vi "AIT 664 - Add Data Channel.vi"(8 "error in (no error)":errorcluster, 11 "Node Ptr":u64 format="%.0x") -> (0 "error out":errorcluster)   [LabVIEW 2013, in "AIT 664 Custom Device.lvlib"]
doc: "Adds a single data channel to a 664 port"
uses:
  AIT 664 Custom Device.lvlib
  <vilib>/NI Veristand/Custom Device API/Custom Device Channel.ctl
  <vilib>/NI Veristand/Custom Device API/Custom Device Channel Type.ctl
  Controls/664 -Param.ctl
  Controls and Global/Global.vi
  <vilib>/NI Veristand/Custom Device API/Get Item Property (U32).vi
  <vilib>/NI Veristand/Custom Device API/Get Item Property (U32 Array).vi
  <vilib>/NI Veristand/Custom Device API/Get Item Property (Boolean).vi
  <vilib>/NI Veristand/Custom Device API/Custom Device API.lvlib
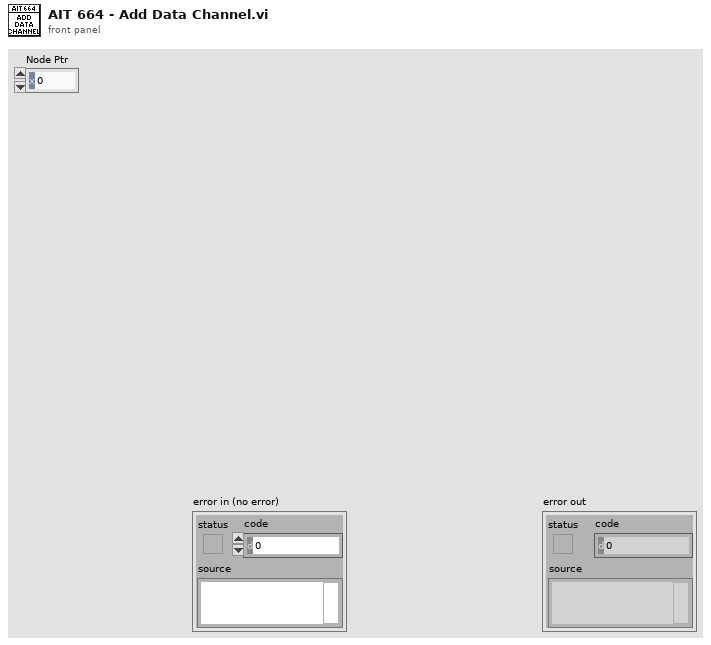
[diagram p1: front panel]
types:
  T1 = typedef "Custom Device API.lvlib/Custom Device Channel Type.ctl" = enum16{"Input", "Output"}
  T2 = typedef "AIT 664 Custom Device.lvlib/664 -Param.ctl" = cluster{"name":string, "firstByte":i32, "startBit":i32, "numberBits":i32, "scaleFactor":dbl, "scaleOffset":dbl, "signed":bool}
  T3 = typedef "Custom Device API.lvlib/Custom Device Channel.ctl" = cluster{"Type":T1, "Units":string, "Default Value":dbl, "Faultable":bool, "Scalable":bool}
  T4 = typedef "Custom Device API.lvlib/Custom Device Item Ref.ctl" = u64
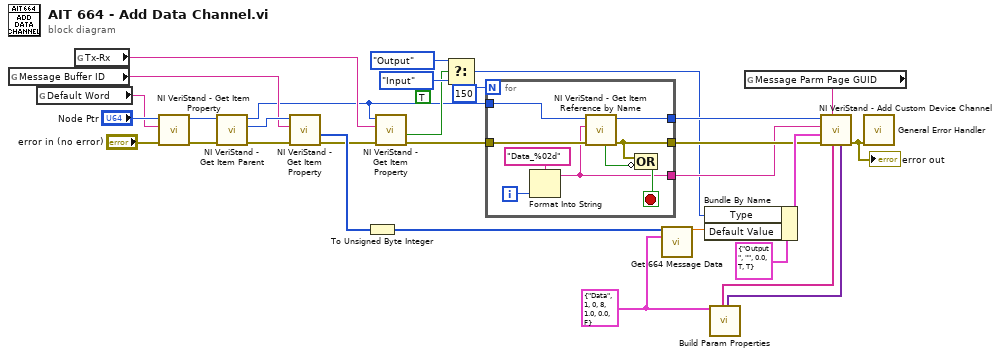
[diagram p0: block diagram]
diagram:
  (unwired) TRUE ("s")
  w9 = T2 {"name"="Data", "firstByte"=1, "startBit"=0, "numberBits"=8, "scaleFactor"=1.0, "scaleOffset"=0.0, "signed"=FALSE} ("1553 Parameter")
  n1 = global read "Global.vi" "Message Buffer ID"() -> (w19:string)
  n2 = global read "Global.vi" "Default Word"() -> (w24:string)
  n3 = global read "Global.vi" "Tx-Rx"() -> (w14:string)
  n4 = call-poly <vilib>:"NI VeriStand - Get Item Property.vi"("error in (no error)"="error in (no error)", "Property Name"=w24, "Item Ref in"="Node Ptr") -> ("error out"=w26:errorcluster, "Item Ref out"=w27:T4)  [unwired: 5 in, 2 out]
  n5 = call <vilib>:"NI VeriStand - Get Item Parent.vi"("error in (no error)"=w26, "Item Ref in"=w27) -> ("error out"=w20:errorcluster, "Parent Ref"=w21:T4, "Item Ref out"=w1:T4)  [unwired: 6 in, 1 out]
  n6 = call-poly <vilib>:"NI VeriStand - Get Item Property.vi"("error in (no error)"=w20, "Property Name"=w19, "Item Ref in"=w21) -> ("error out"=w15:errorcluster, "Value"=w18:u32[])  [unwired: 5 in, 2 out]
  n7 = To Unsigned Byte Integer(number=w18) -> (unsigned 8bit integer=w17:u8[])
  n8 = call-poly <vilib>:"NI VeriStand - Get Item Property.vi"("error in (no error)"=w15, "Property Name"=w14, "Item Ref in"=w1) -> ("error out"=w8:errorcluster, "Value"=w2:bool)  [unwired: 5 in, 2 out]
  n9 = Select(t=Custom_Device_Channel_Type."Output" ("Type"), s=w2, f=Custom_Device_Channel_Type."Input" ("Type")) -> (s? t:f=w3:T1)
  n10 = for {
    N: 150 -> [_]
    tunnel: w1 -> [w39]
    tunnel: w8 -> [w38]
    tunnel: [w36] -> w7
    tunnel: [w34] -> w6
    tunnel: [w31] -> w5
    i -> [w33]
    stop <- w37 stop-if-true
    n11 = Format Into String(format string="Data_%02d" ("name"), w33) -> (resulting string=w31:string)  [unwired: 2 in, 1 out]
    n12 = call <vilib>:"NI VeriStand - Get Item Reference by Name.vi"("error in (no error)"=w38, "Item Name"=w31, "Parent Ref in"=w39) -> ("error out"=w36:errorcluster, "Parent Ref out"=w34:T4, "Found"=w35:bool)  [unwired: 5 in, 1 out]
    n13 = Compound Arithmetic op=OR(w36, invert w35) -> (w37:bool)
  }
  n14 = call "Get 664 Message Data.vi"("MSG DATA"=w17, "664 Parameter"=w9) -> ("Value"=w16:dbl)  [unwired: 12 in, 1 out]
  n15 = Bundle By Name(cluster=T3 {"Type"=enum."Output", "Units"="", "Default Value"=0.0, "Faultable"=TRUE, "Scalable"=TRUE} ("Channel"), "Type"=w3, "Default Value"=w16) -> (w10:T3)
  n16 = call "Build Param Properties.vi"("Parameter"=w9) -> ("Prop Names"=w23:string[], "Prop Values"=w22:variant[])  [unwired: 10 in, 7 out]
  n17 = global read "Global.vi" "Message Parm Page GUID"() -> (w30:string)
  n18 = call <vilib>:"NI VeriStand - Add Custom Device Channel.vi"("Property Values"=w22, "Property names"=w23, "GUID (Default Channel)"=w30, "error in (no error)"=w7, "Channel"=w10, "Channel Name"=w5, "Parent Ref in"=w6) -> ("error out"=w29:errorcluster)  [unwired: 1 in, 3 out]
  "error out" <- w29
  n19 = call <vilib>:"General Error Handler.vi"("error in (no error)"=w29) -> ()  [unwired: 10 in, 5 out]
